vi "Limit factor to PSA.vi"(7 "Input Array":dbl[][](array[numeric]), 8 "error in (no error)":errorcluster, 9 "Number of Columns":i32=2, 10 "Number of Rows":i32=9, 11 "VISA in":refnum<visa-resource-name>) -> (0 "VISA out":refnum<visa-resource-name>, 1 "Numeric2":dbl format="%#_13g", 2 "Numeric1":dbl format="%#_13g", 3 "Resulting string":string)   [LabVIEW 2016]
doc: "Write SCPI commands to PSA to set up limit line."
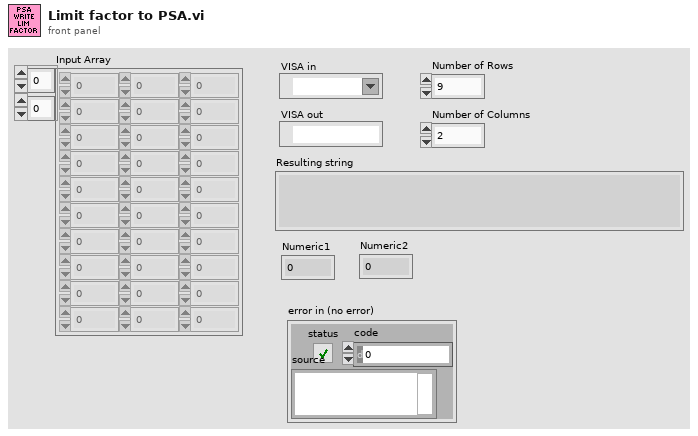
[diagram p1: front panel]
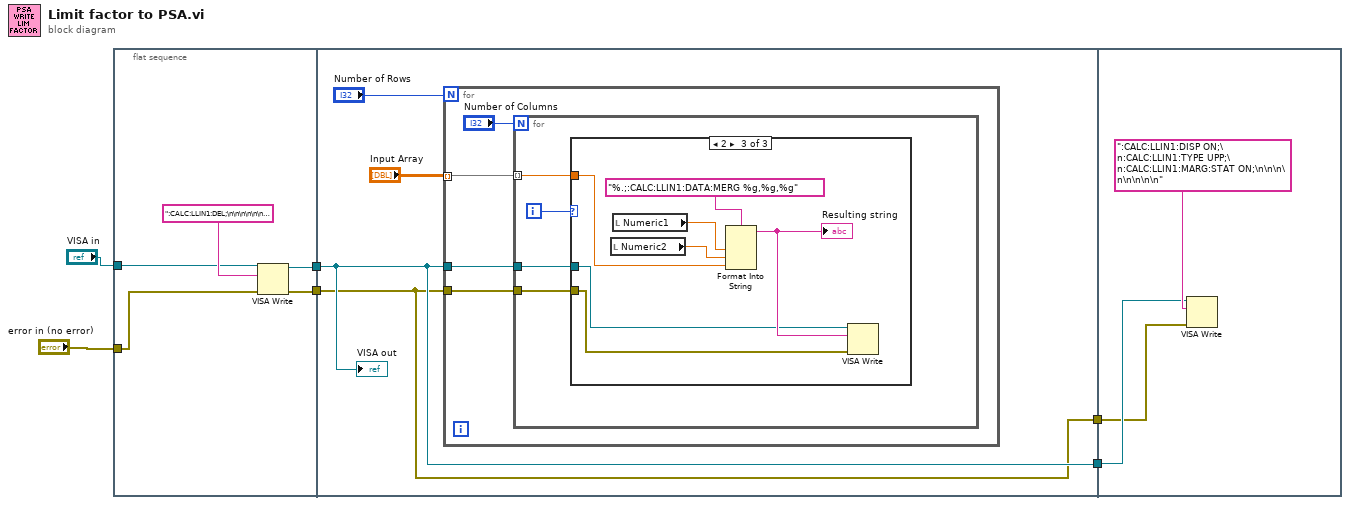
[diagram p0: block diagram]
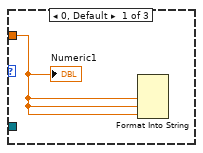
[diagram p2: hidden frame]
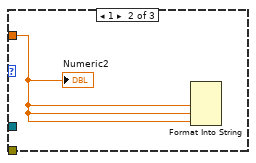
[diagram p3: hidden frame]
diagram:
  n1 = flat-sequence {
    tunnel: [w10] -> w6
    tunnel: [w9] -> w5
    tunnel: "VISA in" -> [w8]
    tunnel: "error in (no error)" -> [w7]
    tunnel: w6 -> [w14]
    tunnel: w5 -> [w13]
    tunnel: [w14] -> w2
    tunnel: [w13] -> w1
    tunnel: w2 -> [w34]
    tunnel: w1 -> [w33]
    frame #0 {
      n2 = VISA Write(VISA resource name=w8, write buffer=":CALC:LLIN1:DEL;\n\n\n\n\n\n\n\n", error in (no error)=w7) -> (VISA resource name out=w10:refnum<visa-resource-name>, error out=w9:errorcluster)  [unwired: 1 out]
    }
    frame #1 {
      n3 = for {
        N: "Number of Rows" -> [_]
        tunnel: "Input Array" -> [w18] mode=indexing
        tunnel: w14 -> [w17]
        tunnel: w13 -> [w16]
        n4 = for {
          N: "Number of Columns" -> [_]
          tunnel: w18 -> [w22] mode=indexing
          tunnel: w17 -> [w21]
          tunnel: w16 -> [w20]
          i -> [w23]
          n5 = case shown="2" w23 {
            tunnel: w22 -> [w24 w25 w26]
            tunnel: w21 -> [_ _ w29]
            tunnel: w20 -> [_ _ w28]
            frame 0, Default {
              n6 = Format Into String(w24, w24, w24) -> ()  [unwired: 3 in, 2 out]
              "Numeric1" <- w24
            }
            frame 1 {
              n7 = Format Into String(w25, w25, w25) -> ()  [unwired: 3 in, 2 out]
              "Numeric2" <- w25
            }
            frame 2 {
              n8 = local read "Numeric2"() -> (w27:dbl)
              n9 = local read "Numeric1"() -> (w31:dbl)
              n10 = Format Into String(format string="%.;:CALC:LLIN1:DATA:MERG %g,%g,%g", w31, w27, w26) -> (resulting string=w30:string)  [unwired: 2 in, 1 out]
              "Resulting string" <- w30
              n11 = VISA Write(VISA resource name=w29, write buffer=w30, error in (no error)=w28) -> ()  [unwired: 3 out]
            }
          }
        }
      }
      "VISA out" <- w14
    }
    frame #2 {
      n12 = VISA Write(VISA resource name=w34, write buffer=":CALC:LLIN1:DISP ON;\n:CALC:LLIN1:TYPE UPP;\n:CALC:LLIN1:MARG:STAT ON;\n\n\n\n\n\n\n\n", error in (no error)=w33) -> ()  [unwired: 3 out]
    }
  }
